vi "Get Window Width.vi"(0 "VI in":refnum<vi>, 11 "error in (no error)":errorcluster) -> (4 "VI out":refnum<vi>, 8 "Width":i16, 15 "error out":errorcluster)   [LabVIEW 2020]
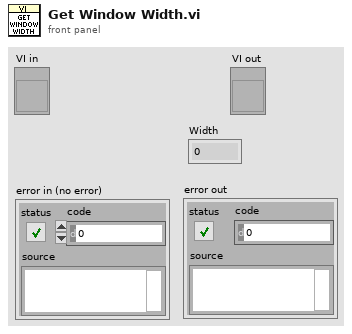
[diagram p1: front panel]
types:
  T1 = typedef "LVRectTypeDef.ctl" = cluster{"Left":i16, "Top":i16, "Right":i16, "Bottom":i16}
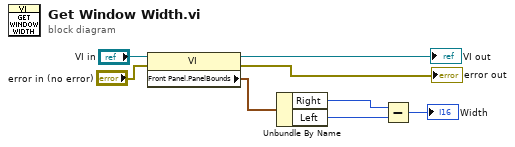
[diagram p0: block diagram]
diagram:
  n1 = property class="VI"(reference="VI in", error in="error in (no error)") -> (reference out=→"VI out":refnum<vi>, error out=→"error out":errorcluster, "Front Panel.PanelBounds"=w8:T1)
  n2 = Unbundle By Name(w8) -> ("Right"=w2:i16, "Left"=w4:i16)
  n3 = Subtract(x=w2, y=w4) -> (x-y=→"Width":i16)
